vi "HILswitch.vi"(7 "u_HIL":dbl[](array[numeric]), 10 "QTM":dbl[](array[numeric])) -> (1 "psi":dbl, 2 "y":dbl, 3 "x":dbl)   [LabVIEW 2014]
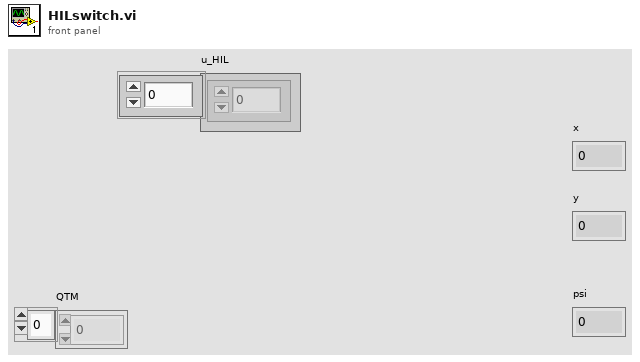
[diagram p1: front panel]
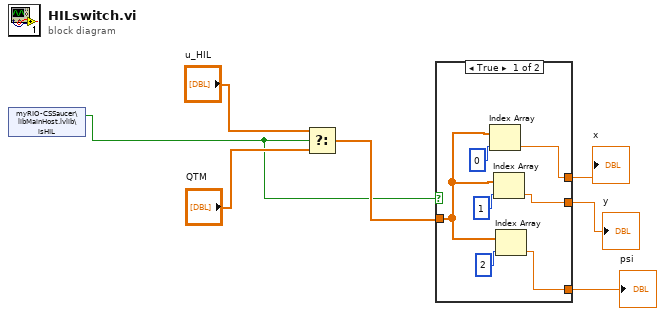
[diagram p0: block diagram]
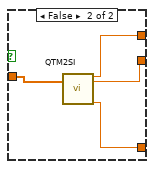
[diagram p2: hidden frame]
diagram:
  n1 = shared-variable "myRIO-CSSaucer\\libMainHost.lvlib\\isHIL"() -> (w1:bool)  [unwired: 1 in, 1 out]
  n2 = Select(t="u_HIL", s=w1, f="QTM") -> (s? t:f=w5:dbl[])
  n3 = case shown="True" w1 {
    tunnel: w5 -> [w11 w18]
    tunnel: [w10 w17] -> w3
    tunnel: [w9 w16] -> w4
    tunnel: [w8 w15] -> w2
    frame True {
      n4 = Index Array(array=w11, index=0) -> (element=w10:dbl)
      n5 = Index Array(array=w11, index=1) -> (element=w9:dbl)
      n6 = Index Array(array=w11, index=2) -> (element=w8:dbl)
    }
    frame False {
      n7 = call "QTM2SI.vi"("Array"=w18) -> ("x"=w17:dbl, "y"=w16:dbl, "psi"=w15:dbl)  [unwired: 13 in, 3 out]
    }
  }
  "y" <- w4
  "x" <- w3
  "psi" <- w2
